vi "setMaxVelo.vi"(8 "error in (no error)":errorcluster, 9 "NewVal":dbl, 10 "Settings":T1={"max velocity"={"Value"=0.0, "Min"=0.0, "Max"=0.0, "StepSize"=0.0, "Tolerance"=0.0, "valueactual"=0.0}, "continious velocity"={"Value"=0.0, "Min"=0.0, "Max"=0.0, "StepSize"=0.0, "Tolerance"=0.0, "valueactual"=0.0}, "shake"=enum."off", "direction"=enum."left", "RedRatio"={"Value"=0.0, "Min"=0.0, "Max"=0.0, "StepSize"=0.0, "Tolerance"=0.0, "valueactual"=0.0}, "StepSize"={"Value"=0.0, "Min"=0.0, "Max"=0.0, "StepSize"=0.0, "Tolerance"=0.0, "valueactual"=0.0}, "position"={"Value"=0.0, "Min"=0.0, "Max"=0.0, "StepSize"=0.0, "Tolerance"=0.0, "valueactual"=0.0}, "velocity"={"Value"=0.0, "Min"=0.0, "Max"=0.0, "StepSize"=0.0, "Tolerance"=0.0, "valueactual"=0.0}, "Step"=enum."off", "Mode"=enum."on demand", "timeout"={"Value"=0.0, "Min"=0.0, "Max"=0.0, "StepSize"=0.0, "Tolerance"=0.0, "valueactual"=0.0}, "DelayStage"={"Value"=0.0, "Min"=0.0, "Max"=0.0, "StepSize"=0.0, "Tolerance"=0.0, "valueactual"=0.0}, "TapeMotor"=enum."off", "encoder Axis"=2, "oldpos"=0.0, "ResetEncoder"=enum."off"}, 11 "VISA Refnum in":refnum<visa-resource-name>) -> (0 "error out":errorcluster, 1 "max velocity.Value":dbl, 2 "Settings":T1={"max velocity"={"Value"=0.0, "Min"=0.0, "Max"=0.0, "StepSize"=0.0, "Tolerance"=0.0, "valueactual"=0.0}, "continious velocity"={"Value"=0.0, "Min"=0.0, "Max"=0.0, "StepSize"=0.0, "Tolerance"=0.0, "valueactual"=0.0}, "shake"=enum."off", "direction"=enum."left", "RedRatio"={"Value"=0.0, "Min"=0.0, "Max"=0.0, "StepSize"=0.0, "Tolerance"=0.0, "valueactual"=0.0}, "StepSize"={"Value"=0.0, "Min"=0.0, "Max"=0.0, "StepSize"=0.0, "Tolerance"=0.0, "valueactual"=0.0}, "position"={"Value"=0.0, "Min"=0.0, "Max"=0.0, "StepSize"=0.0, "Tolerance"=0.0, "valueactual"=0.0}, "velocity"={"Value"=0.0, "Min"=0.0, "Max"=0.0, "StepSize"=0.0, "Tolerance"=0.0, "valueactual"=0.0}, "Step"=enum."off", "Mode"=enum."on demand", "timeout"={"Value"=0.0, "Min"=0.0, "Max"=0.0, "StepSize"=0.0, "Tolerance"=0.0, "valueactual"=0.0}, "DelayStage"={"Value"=0.0, "Min"=0.0, "Max"=0.0, "StepSize"=0.0, "Tolerance"=0.0, "valueactual"=0.0}, "TapeMotor"=enum."off", "encoder Axis"=2, "oldpos"=0.0, "ResetEncoder"=enum."off"}, 3 "VISA Refnum out":refnum<visa-resource-name>)   [LabVIEW 2011]
uses:
  TapeDrive/settings_TypDef.ctl
  shared/numericVariable_TypeDef.ctl
  shared/OnOffTypeDef.ctl
  TapeDrive/Direction_TypDef.ctl
  TapeDrive/Mode_TypDEf.ctl
  <instrlib>/Newport ESP301/Newport ESP301.lvlib
  TapeDrive/TapeDrive.lvclass
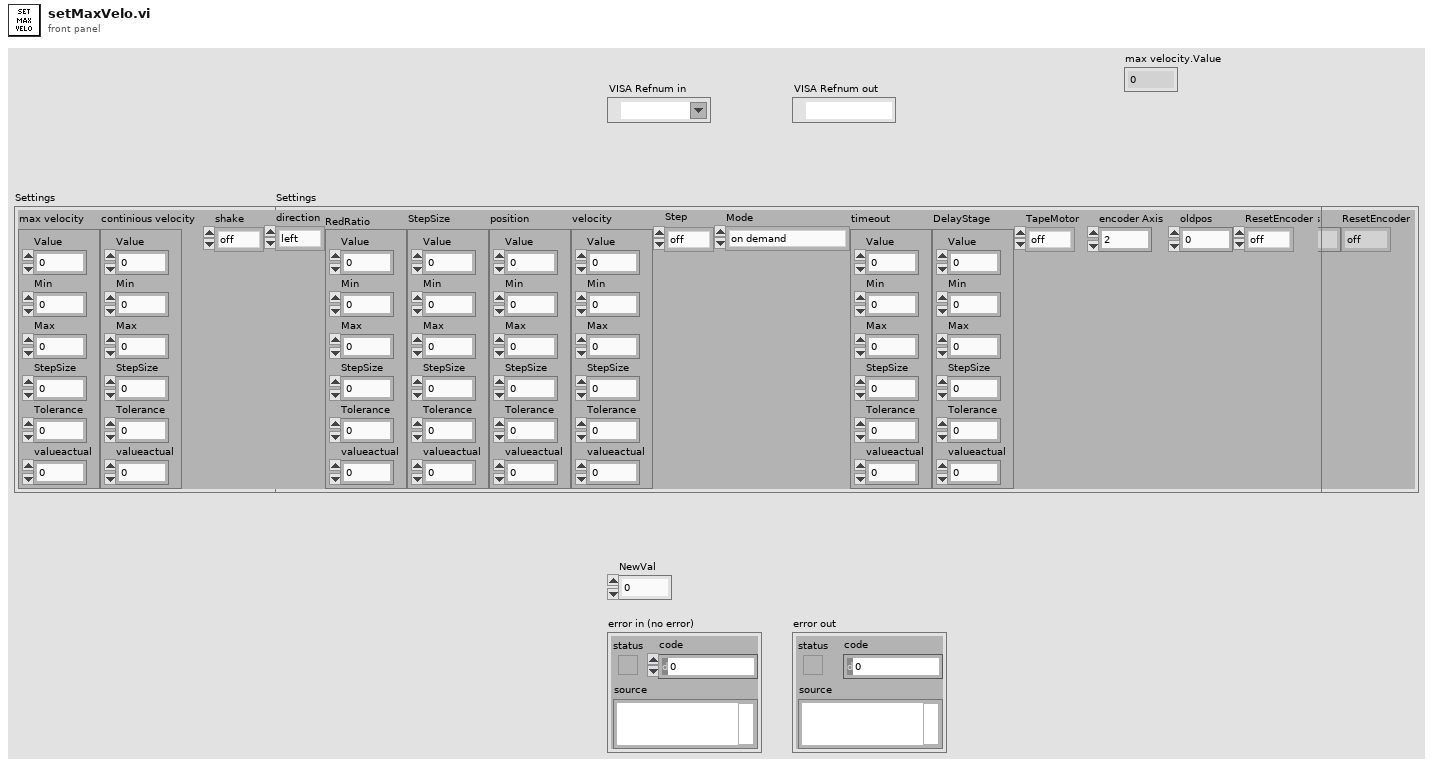
[diagram p1: front panel]
types:
  T1 = typedef "TapeDrive.lvclass/settings_TypDef.ctl" = cluster{"max velocity":T2, "continious velocity":T2, "shake":T3, "direction":T4, "RedRatio":T2, "StepSize":T2, "position":T2, "velocity":T2, "Step":T3, "Mode":T5, "timeout":T2, "DelayStage":T2, "TapeMotor":T3, "encoder Axis":i32, "oldpos":dbl, "ResetEncoder":T3}
  T2 = typedef "numericVariable_TypeDef.ctl" = cluster{"Value":dbl, "Min":dbl, "Max":dbl, "StepSize":dbl, "Tolerance":dbl, "valueactual":dbl}
  T3 = typedef "OnOffTypeDef.ctl" = enum16{"off", "on"}
  T4 = typedef "Direction_TypDef.ctl" = enum16{"left", "right"}
  T5 = typedef "Mode_TypDEf.ctl" = enum16{"on demand", "continuous", "scan"}
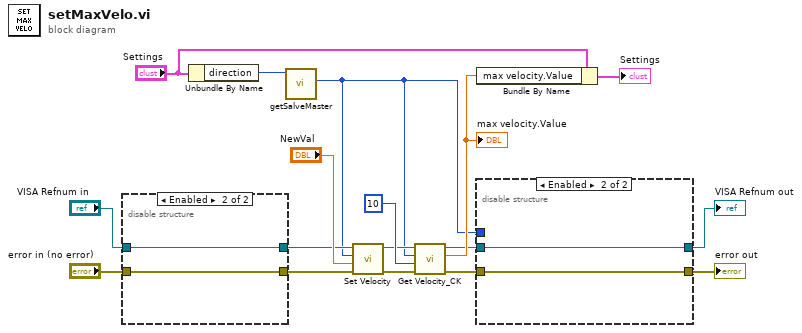
[diagram p0: block diagram]
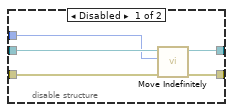
[diagram p2: hidden frame]
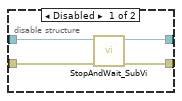
[diagram p3: hidden frame]
diagram:
  n1 = disable-structure shown="Enabled" {
    disable-tunnel: "VISA Refnum in" -> [w21 w23]
    disable-tunnel: [w20 w23] -> w8
    disable-tunnel: "error in (no error)" -> [w19 w22]
    disable-tunnel: [w18 w22] -> w1
    frame Disabled {
      n2 = call "StopAndWait_SubVi.vi"("error in (no error)"=w19, "VISA Refnum in"=w21) -> ("error out"=w18:errorcluster, "VISA Refnum out"=w20:refnum<visa-resource-name>)  [unwired: 8 in]
    }
    frame Enabled {
    }
  }
  n3 = Unbundle By Name("Settings") -> ("direction"=w15:T4)
  n4 = call "getSalveMaster.vi"("direction"=w15) -> ("Master"=w2:i32)  [unwired: 9 in, 1 out]
  n5 = call <instrlib>:"Set Velocity.vi"("error in (no error)"=w1, "Velocity (units/s)"="NewVal", "Axis (1)"=w2, "VISA resource name"=w8) -> ("error out"=w14:errorcluster, "VISA resource name out"=w12:refnum<visa-resource-name>)  [unwired: 2 in]
  n6 = call "Get Velocity_CK.vi"("error in (no error)"=w14, "Wait before read (0ms)"=u32 10, "Axis (1)"=w2, "VISA resource name"=w12) -> ("error out"=w4:errorcluster, "Velocity (units/s)"=w10:dbl, "VISA resource name out"=w6:refnum<visa-resource-name>)  [unwired: 1 in]
  "max velocity.Value" <- w10
  n7 = Bundle By Name(cluster="Settings", "max velocity.Value"=w10) -> (→"Settings":T1)
  n8 = disable-structure shown="Enabled" {
    disable-tunnel: w6 -> [w28 w30]
    disable-tunnel: [w27 w30] -> w5
    disable-tunnel: w4 -> [w26 w29]
    disable-tunnel: [w25 w29] -> w3
    disable-tunnel: w2 -> [w24 _]
    frame Disabled {
      n9 = call <instrlib>:"Move Indefinitely.vi"("error in (no error)"=w26, "Axis (1)"=w24, "VISA resource name"=w28) -> ("error out"=w25:errorcluster, "VISA resource name out"=w27:refnum<visa-resource-name>)  [unwired: 3 in]
    }
    frame Enabled {
    }
  }
  "error out" <- w3
  "VISA Refnum out" <- w5
